vi "Prompt for Step.vi"(8 "error in (no error)":errorcluster, 11 "Wait Action in":refnum<class "Wait Action.lvclass">) -> (0 "error out":errorcluster, 2 "OK?":bool, 3 "Wait Action out":refnum<class "Wait Action.lvclass">)   [LabVIEW 2020, in "MacroAssert.lvlib" / "Wait Action.lvclass"]
uses:
  Wait Action.lvclass
  Wait Action.lvclass/Wait Action.ctl
  Action Step/Action Step.lvclass
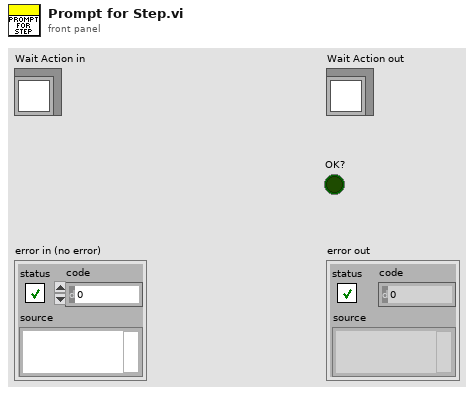
[diagram p1: front panel]
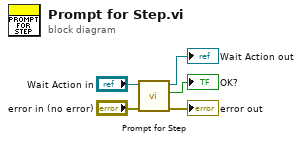
[diagram p0: block diagram]
diagram:
  n1 = call-parent "Prompt for Step.vi"("error in (no error)"="error in (no error)", "Step in"="Wait Action in") -> ("error out"=→"error out":errorcluster, "OK?"=→"OK?":bool, "Step out"=→"Wait Action out":refnum<class "Wait Action.lvclass">)  [unwired: 7 in]
